vi "Count Down.vi"(8 "error in":errorcluster, 9 "preset value":u32=10, 10 "load":bool, 11 "count down":bool) -> (0 "error out":errorcluster, 2 "counter value":u32, 3 "done":bool)   [LabVIEW 2020, in "NI_FunctionBlock Libraries.lvlib"]
uses:
  <vilib>/functionblocks/NI_FunctionBlock Libraries.lvlib
  <vilib>/ptbypt/NI_PtbyPt.lvlib
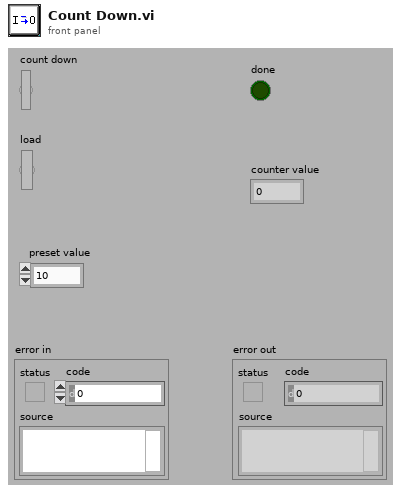
[diagram p1: front panel]
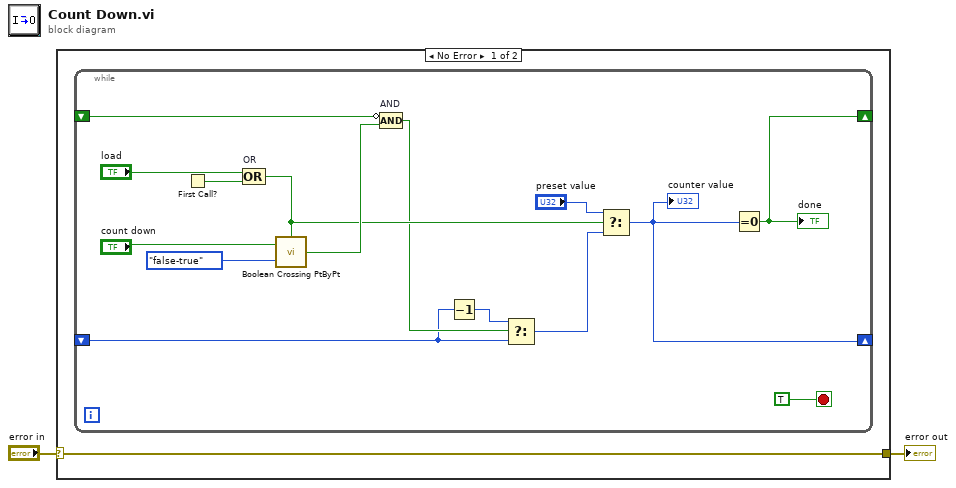
[diagram p0: block diagram]
diagram:
  n1 = case shown="No Error" "error in" {
    selector: "error in" -> [w3 w19]
    tunnel: [w3 w19] -> w1
    frame No Error {
      n2 = while {
        shift-right: [w12] -> _
        shift-left: _ -> [w13]
        shift-right: [w6] -> _
        shift-left: _ -> [w7]
        stop <- TRUE stop-if-true
        n3 = First Call?() -> (First Call?: T/F=w15:bool)
        n4 = Compound Arithmetic op=OR "OR"("load", w15) -> (w9:bool)
        n5 = call <vilib>:"Boolean Crossing PtByPt.vi"("initialize"=w9, "direction"=enum16{"either", "false-true", "true-false"}."false-true", "input"="count down") -> ("crossing"=w11:bool)
        n6 = Compound Arithmetic op=AND "AND"(invert w13, w11) -> (w8:bool)
        n7 = Decrement(x=w7) -> (x-1=w5:u32)
        n8 = Select(t=w5, s=w8, f=w7) -> (s? t:f=w4:u32)
        n9 = Select(t="preset value", s=w9, f=w4) -> (s? t:f=w6:u32)
        "counter value" <- w6
        n10 = Equal To 0?(x=w6) -> (x = 0?=w12:bool)
        "done" <- w12
      }
    }
    frame Error {
    }
  }
  "error out" <- w1
